vi "自适应屏幕分辨率.vi"(1 "error in (no error)":errorcluster) -> (0 "error out":errorcluster)   [LabVIEW 2019]
panel:
  # "www.vihome.com.cn\nby iwanttofly"
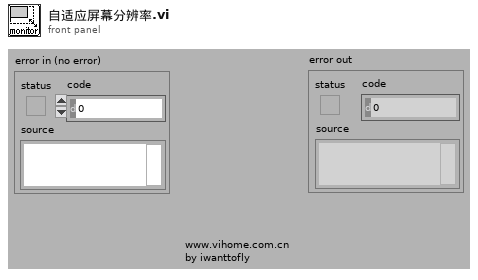
[diagram p1: front panel]
types:
  T1 = typedef "LVPointTypeDef.ctl" = cluster{"Horizontal":i16, "Vertical":i16}
  T2 = typedef "LVRectTypeDef.ctl" = cluster{"Left":i16, "Top":i16, "Right":i16, "Bottom":i16}
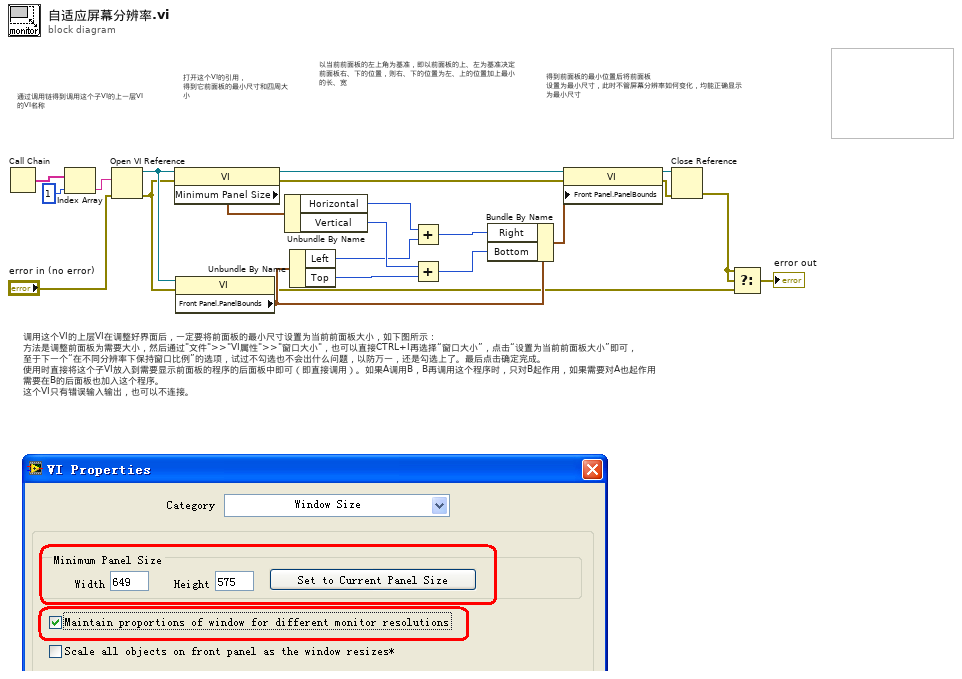
[diagram p0: block diagram]
diagram:
  # "调用这个VI的上层VI在调整好界面后，一定要将前面板的最小尺寸设置为当前前面板大小，如下图所示：\n方法是调整前面板为需要大小，然后通过\"文件\">>\"VI属性\">>\"窗口大小\"，也可以直接CTRL+I再选择“窗口大小”，点击“设置为当前前面板大小”即可，\n至于下一个“在不同分辨率下保持窗口比例”的选项，试过不勾选也不会出什么问题，以防万一，还是勾选上了。最后点击确定完成。\n使用时直接将这个子VI放入到需要显示前面板的程序的后面板中即可（即直接调用）。如果A调用B，B再调用这个程序时，只对B起作用，如果需要对A也起作用\n需要在B的后面板也加入这个程序。\n这个VI只有错误输入输出，也可以不连接。"
  # "得到前面板的最小位置后将前面板\n设置为最小尺寸，此时不管屏幕分辨率如何变化，均能正确显示为最小尺寸"
  # "以当前前面板的左上角为基准，即以前面板的上、左为基准决定前面板右、下的位置，则右、下的位置为左、上的位置加上最小的长、宽"
  # "打开这个VI的引用，\n得到它前面板的最小尺寸和四周大小"
  # "通过调用链得到调用这个子VI的上一层VI的VI名称"
  n1 = Call Chain ("调用链")() -> (call chain=w19:string[])
  n2 = Index Array(array=w19, index=1) -> (element=w21:string)
  n3 = Open VI Reference(vi path=w21, error in (no error)="error in (no error)") -> (vi reference=w18:refnum<vi>, error out=w2:errorcluster)  [unwired: 4 out]
  n4 = property class="VI"(reference=w18, error in=w2) -> (reference out=w22:refnum<vi>, error out=w8:errorcluster, "Minimum Panel Size"=w17:T1)
  n5 = property class="VI"(reference=w18, error in=w2) -> (error out=w6:errorcluster, "Front Panel.PanelBounds"=w11:T2)  [unwired: 1 out]
  n6 = Unbundle By Name(w17) -> ("Horizontal"=w10:i16, "Vertical"=w13:i16)
  n7 = Unbundle By Name(w11) -> ("Left"=w9:i16, "Top"=w14:i16)
  n8 = Add(x=w10, y=w9) -> (x+y=w12:i16)
  n9 = Add(x=w13, y=w14) -> (x+y=w15:i16)
  n10 = Bundle By Name(cluster=w11, "Right"=w12, "Bottom"=w15) -> (w16:T2)
  n11 = property class="VI"(reference=w22, error in=w8, "Front Panel.PanelBounds"=w16) -> (reference out=w5:refnum<vi>, error out=w4:errorcluster)
  n12 = Close Reference(reference=w5, error in (no error)=w4) -> (error out=w3:errorcluster)
  n13 = Select(t=w3, s=w3, f=w6) -> (s? t:f=→"error out":errorcluster)
